vi "Global Log To String(Periodic Check).vi"(0 "Cross CSM Data":T3, 1 "Reset?":bool, 2 "Remove Immediately? (F)":bool, 3 "Time Format String":string="%<%H:%M:%S%3u>T", 9 "Settings":T2={"threashold(#/s)"=1.9, "Check Peroid(s)"=1.0}, 12 "Level (Normal)":T1) -> (4 "String":string, 10 "Periodic Info":string[](array[string]))   [LabVIEW 2017, in "Communicable State Machine.lvlib"]
uses:
  Communicable State Machine.lvlib
  _Support/Typedef/_CSM_GlobalLog_MSG.ctl
  _Support/Typedef/_CSM_Response Source Message.ctl
  _Support/Typedef/_CSM_GlobalLog_MSG_TYPE.ctl
  Periodic String Filter Setting.ctl
  _support/Periodic String Filter Level.ctl
  Periodic String Filter State.ctl
  _Shared/CSM Shared.lvlib
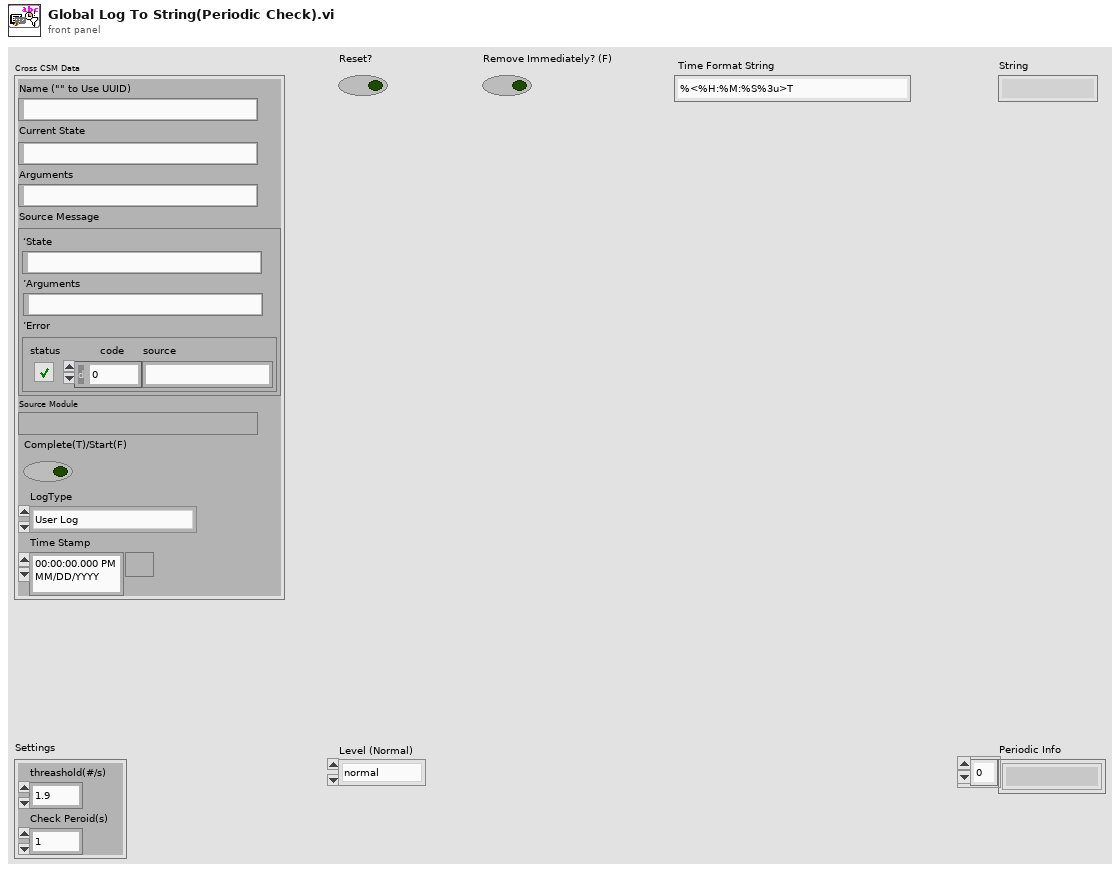
[diagram p1: front panel]
types:
  T1 = typedef "Communicable State Machine.lvlib/Periodic String Filter Level.ctl" = enum16{"normal", "L1", "L2", "L3", "L4"}
  T2 = typedef "Communicable State Machine.lvlib/Periodic String Filter Setting.ctl" = cluster{"threashold(#/s)":dbl, "Check Peroid(s)":dbl}
  T3 = typedef "Communicable State Machine.lvlib/_CSM_GlobalLog_MSG.ctl" = cluster{"Name (\"\" to Use UUID)":string, "Current State":string, "Arguments":string, "Source Message":T4, "Source Module":string, "Complete(T)/Start(F)":bool, "LogType":T5, "Time Stamp":timestamp}
  T4 = typedef "Communicable State Machine.lvlib/_CSM_Response Source Message.ctl" = cluster{"‘State":string, "’Arguments":string, "’Error":errorcluster}
  T5 = typedef "Communicable State Machine.lvlib/_CSM_GlobalLog_MSG_TYPE.ctl" = enum16{"User Log", "State Change", "Status", "Interrupt", "Register", "Unregister", "Error Log", "Module Created", "Module Destroyed", "Async Message", "No-Rep Async Message", "Sync Message"}
  T6 = typedef "Communicable State Machine.lvlib/Periodic String Filter State.ctl" = enum16{"Normal", "Remove All Filters"}
  T7 = typedef "Communicable State Machine.lvlib/Periodic String Filter Data.ctl" = cluster{"Keys":string[], "Count":i64[], "LastCheckT":timestamp[], "LastCheckN":i64[], "Filtered":cluster{"Keys":string[], "StartingCount":i64[], "entry":T8[]}}
  T8 = typedef "Communicable State Machine.lvlib/Periodic String Filter Info.ctl" = cluster{"String":string, "Count":i64, "since":timestamp, "param":string, "speed":dbl}
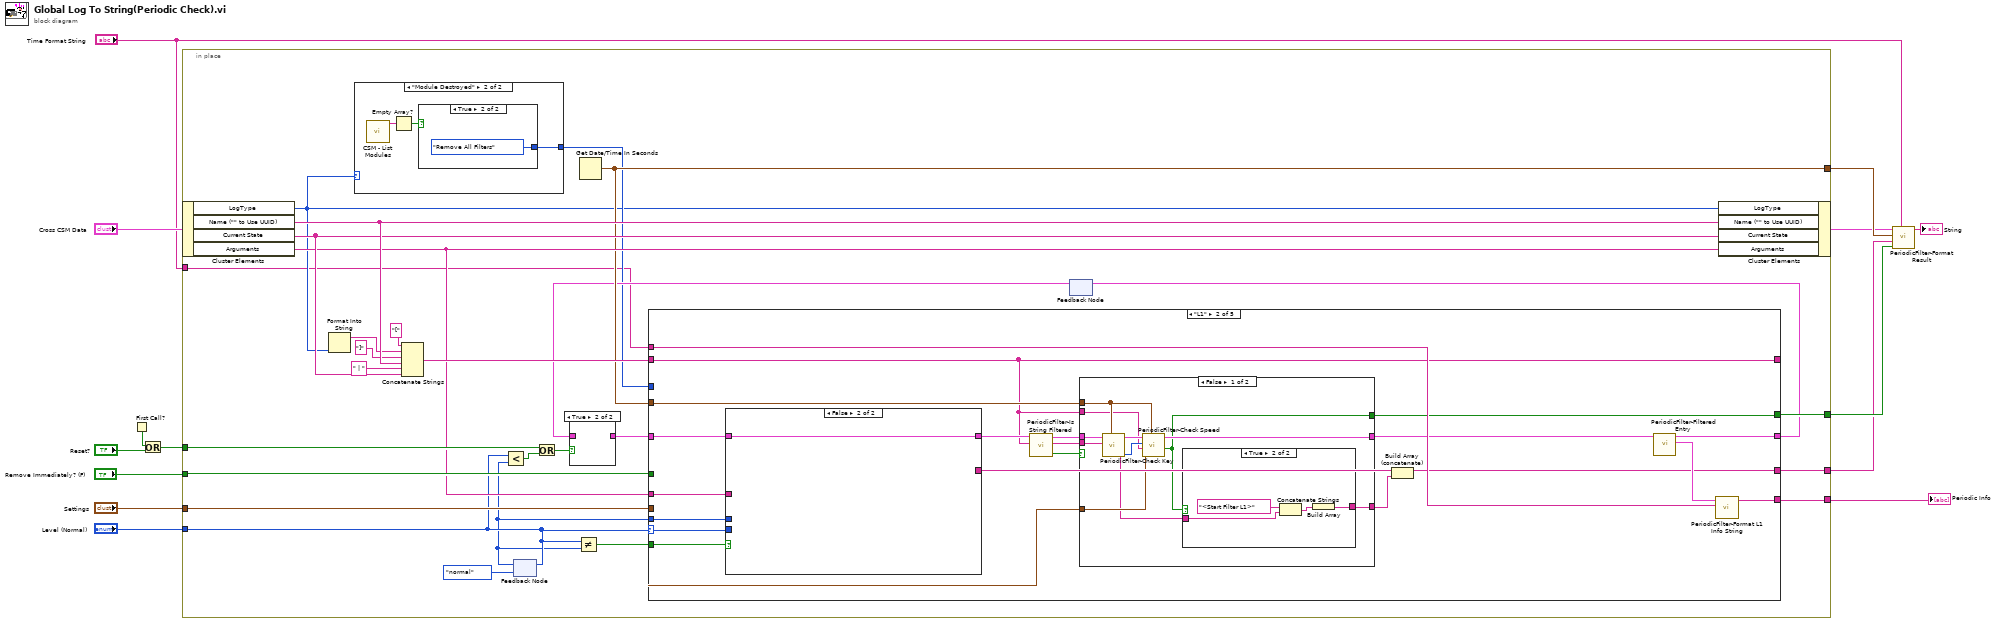
[diagram p0: block diagram]
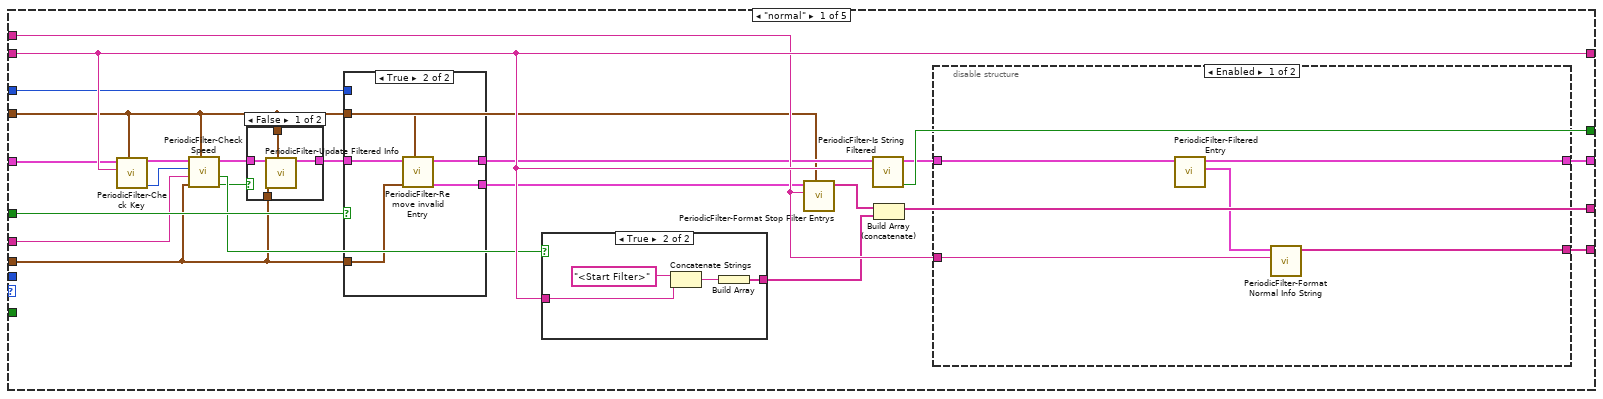
[diagram p4: hidden frame]
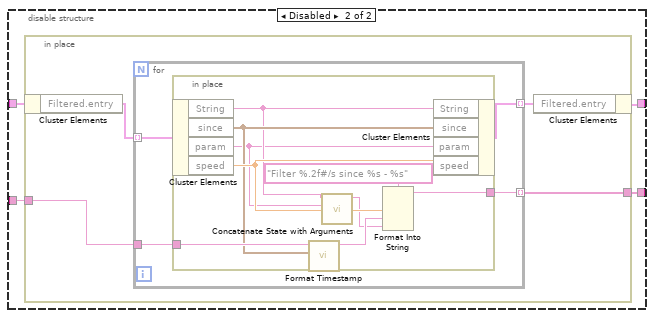
[diagram p6: hidden frame]
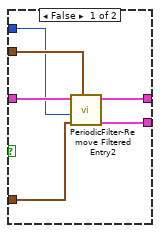
[diagram p7: hidden frame]
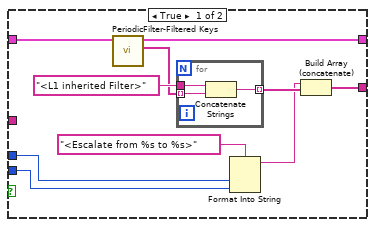
[diagram p11: hidden frame]
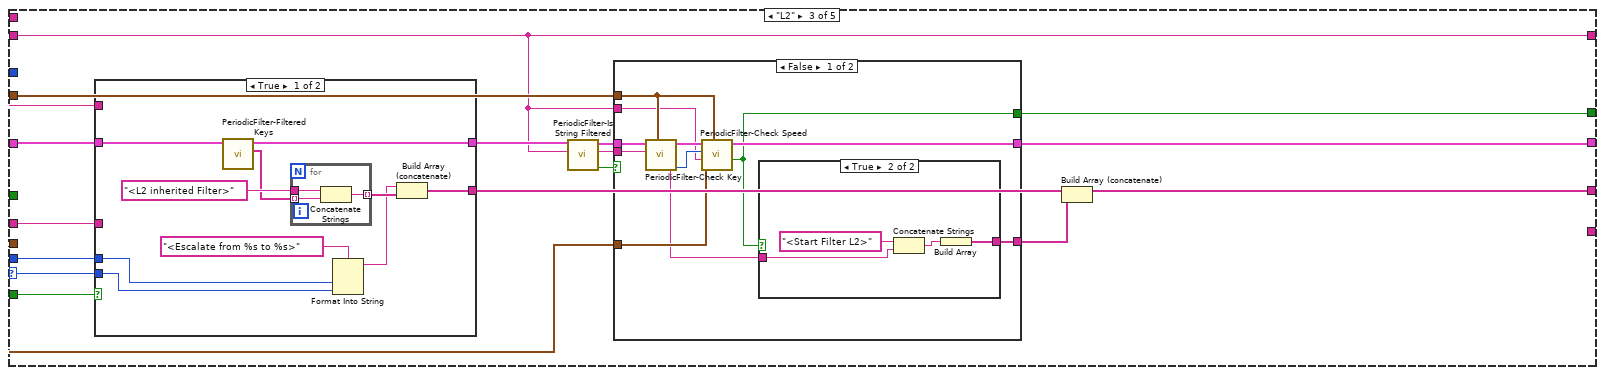
[diagram p12: hidden frame]
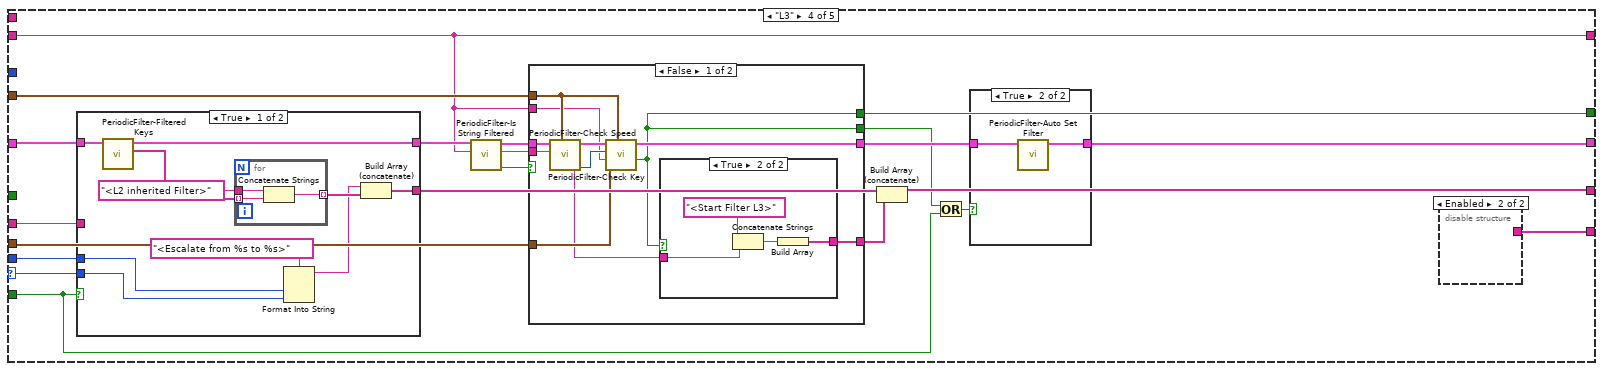
[diagram p16: hidden frame]
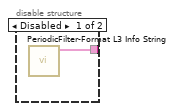
[diagram p17: hidden frame]
diagram:
  n1 = First Call?() -> (First Call?: T/F=w5:bool)
  n2 = Or(x=w5, y="Reset?") -> (x .or. y?=w6:bool)
  n3 = in-place "In Place Element Structure" {
    in-place-border: w6 -> [w38]
    in-place-border: [w36] -> w10
    in-place-border: "Remove Immediately? (F)" -> [w33]
    in-place-border: "Settings" -> [w32]
    in-place-border: "Level (Normal)" -> [w16]
    in-place-border: [w29] -> w9
    in-place-border: [w19] -> w1
    in-place-border: [w18] -> w4
    in-place-border: "Time Format String" -> [w17]
    n4 = in-place-cluster #1("Cross CSM Data") -> ("LogType"=w20:T5, "Name (\"\" to Use UUID)"=w41:string, "Current State"=w40:string, "Arguments"=w31:string)
    n5 = Format Into String(w20) -> (resulting string=w30:string)  [unwired: 3 in, 1 out]
    n6 = case shown="\"Module Destroyed\"" w20 {
      tunnel: [_ w42] -> w21
      frame "User Log", Default {
      }
      frame "Module Destroyed" {
        n7 = call "CSM - List Modules.vi"() -> ("Module Names"=w44:string[])  [unwired: 10 in, 1 out]
        n8 = Empty Array?(array=w44) -> (empty?=w43:bool)
        n9 = case shown="True" w43 {
          tunnel: [_ Periodic_String_Filter_State."Remove All Filters" ("State")] -> w42
          frame False {
          }
          frame True {
          }
        }
      }
    }
    n10 = Concatenate Strings("[" ("string"), w30, "]" ("string"), w41, " | " ("string"), w40) -> (w37:string)
    n11 = feedback #2(Periodic_String_Filter_Level."normal" ("Level(Normal)")) -> (w15:T1)
    n12 = Less?(x=w16, y=w15) -> (x < y?=w27:bool)
    n13 = feedback-in #2(w16) -> ()
    n14 = Or(x=w38, y=w27) -> (x .or. y?=w22:bool)
    n15 = Not Equal?(x=w16, y=w15) -> (x != y?=w26:bool)
    n16 = Get Date/Time In Seconds() -> (seconds since 1Jan1904=w29:timestamp)
    n17 = feedback #3() -> (w25:T7)  [unwired: 1 in]
    n18 = case shown="True" w22 {
      tunnel: [w278 _] -> w24
      tunnel: w25 -> [w278 _]
      frame False {
      }
      frame True {
      }
    }
    n19 = case shown="\"L1\"" w16 {
      selector: w16 -> [_ w115 w166 w213 _]
      tunnel: w37 -> [w68 w117 w168 w220 w273]
      tunnel: [w68 w117 w168 w220 w273] -> _
      tunnel: w32 -> [w48 w121 w172 w223 _]
      tunnel: w29 -> [w46 w122 w173 w224 _]
      tunnel: [w66 w128 w175 w219 w269] -> w23
      tunnel: w24 -> [w65 w135 w182 w233 w271]
      tunnel: [w64 w120 w171 w217 TRUE ("new filtered Item")] -> w36
      tunnel: w33 -> [w67 _ _ _ _]
      tunnel: w26 -> [_ w134 w181 w218 w270]
      tunnel: w31 -> [w63 w133 w180 w232 _]
      tunnel: w21 -> [w62 _ _ _ _]
      tunnel: [w61 w132 _ w231 _] -> w19
      tunnel: [w60 w119 w170 w222 w268] -> w18
      tunnel: w17 -> [w59 w131 _ _ _]
      tunnel: w15 -> [_ w116 w167 w214 _]
      frame "normal" {
        n20 = call "PeriodicFilter-Check Key.vi"("Seconds Since 1Jan1904 2"=w46, "Key"=w68, "Data In"=w65) -> ("Index"=w58:i32, "Data Out"=w57:T7)  [unwired: 7 in]
        n21 = call "PeriodicFilter-Check Speed.vi"("Seconds Since 1Jan1904"=w46, "Settings"=w48, "Parameter"=w63, "Index"=w58, "Data In"=w57) -> ("Over Threshold?"=w47:bool, "New Filtered Item"=w54:bool, "Data Out"=w56:T7)  [unwired: 4 in]
        n22 = case shown="False" w47 {
          tunnel: w56 -> [w72 w73]
          tunnel: [w71 w73] -> w55
          tunnel: w46 -> [w70 _]
          tunnel: w48 -> [w69 _]
          frame False {
            n23 = call "PeriodicFilter-Update Filtered Info.vi"("Seconds Since 1Jan1904"=w70, "Settings"=w69, "Data In"=w72) -> ("Data Out"=w71:T7)  [unwired: 8 in]
          }
          frame True {
          }
        }
        n24 = case shown="True" w67 {
          tunnel: w55 -> [w105 w110]
          tunnel: w46 -> [w104 w109]
          tunnel: [w103 w108] -> w53
          tunnel: [w102 w107] -> w52
          tunnel: w48 -> [w100 w106]
          tunnel: w62 -> [w101 _]
          frame False {
            n25 = call "PeriodicFilter-Remove Filtered Entry2.vi"("Seconds Since 1Jan1904 2"=w104, "Settings"=w100, "State"=w101, "Data In"=w105) -> ("Removed Info"=w102:T8[], "Data Out"=w103:T7)  [unwired: 6 in]
          }
          frame True {
            n26 = call "PeriodicFilter-Remove invalid Entry.vi"("Seconds Since 1Jan1904 2"=w109, "Settings"=w106, "Data In"=w110) -> ("Removed Info"=w107:T8[], "Data Out"=w108:T7)  [unwired: 7 in]
          }
        }
        n27 = case shown="True" w54 {
          tunnel: [_ w114] -> w50
          tunnel: w68 -> [_ w112]
          frame False {
          }
          frame True {
            n28 = Concatenate Strings("<Start Filter>" ("Current State"), w112) -> (w111:string)
            n29 = Build Array(w111) -> (w114:string[])
          }
        }
        n30 = call "PeriodicFilter-Format Stop Filter Entrys.vi"("Seconds Since 1Jan1904 2"=w46, "Time Format String"=w59, "Removed Info"=w52) -> ("Array"=w49:string[])  [unwired: 8 in]
        n31 = call "PeriodicFilter-Is String Filtered.vi"("Input String"=w68, "Data In"=w53) -> ("Filtered"=w64:bool, "Data Out"=w51:T7)  [unwired: 7 in, 1 out]
        n32 = Build Array (concatenate)(w49, w50) -> (w60:string[])
        n33 = disable-structure shown="Enabled" {
          disable-tunnel: [w78 w81] -> w66
          disable-tunnel: [w77 w79] -> w61
          disable-tunnel: w59 -> [w76 w80]
          disable-tunnel: w51 -> [w75 w82]
          frame Enabled {
            n34 = call "PeriodicFilter-Filtered Entry.vi"("Data In"=w75) -> ("Entry"=w74:T8[], "Data Out"=w78:T7)  [unwired: 9 in]
            n35 = call "PeriodicFilter-Format Normal Info String.vi"("Time Format String"=w76, "Removed Info"=w74) -> ("Array"=w77:string[])  [unwired: 9 in]
          }
          frame Disabled {
            n36 = in-place {
              in-place-border: w80 -> [w85]
              in-place-border: [w84] -> w79
              n37 = in-place-cluster #4(w82) -> ("Filtered.entry"=w86:T8[])
              n38 = for {
                tunnel: w86 -> [w88] mode=indexing
                tunnel: [w90] -> w84 mode=indexing
                tunnel: w85 -> [w89]
                tunnel: [w87] -> w83 mode=indexing
                n39 = in-place {
                  in-place-border: [w99] -> w90
                  in-place-border: w89 -> [w96]
                  n40 = in-place-cluster #5(w88) -> ("String"=w93:string, "since"=w94:timestamp, "param"=w91:string, "speed"=w95:dbl)
                  n41 = call "Format Timestamp.vi"("Timestamp"=w94, "Format String"=w96) -> ("String"=w97:string)  [unwired: 9 in]
                  n42 = call "Concatenate State with Arguments.vi"("Arguments"=w91, "State"=w93) -> ("State With Arguements"=w92:string)  [unwired: 9 in]
                  n43 = Format Into String(format string="Filter %.2f#/s since %s - %s", w95, w97, w92) -> (resulting string=w99:string)  [unwired: 2 in, 1 out]
                  n44 = in-place-cluster #5("String"=w93, "since"=w94, "param"=w91, "speed"=w95) -> (w87:T8)
                }
              }
              n45 = in-place-cluster #4("Filtered.entry"=w83) -> (w81:T7)
            }
          }
        }
      }
      frame "L1" {
        n46 = case shown="False" w134 {
          tunnel: w135 -> [w161 w165]
          tunnel: [w156 w165] -> w123
          tunnel: [w157 _] -> w130
          tunnel: w133 -> [_ _]
          tunnel: w116 -> [w154 _]
          tunnel: w115 -> [w153 _]
          frame True {
            n47 = call "PeriodicFilter-Filtered Keys.vi"("Data In"=w161) -> ("Filtered Keys"=w159:string[], "Data Out"=w156:T7)  [unwired: 9 in]
            n48 = for {
              tunnel: w159 -> [w164] mode=indexing
              tunnel: [w163] -> w158 mode=indexing
              tunnel: "<L1 inherited Filter>" ("Current State") -> [w162]
              n49 = Concatenate Strings(w162, w164) -> (w163:string)
            }
            n50 = Format Into String(format string="<Escalate from %s to %s>" ("Current State"), w154, w153) -> (resulting string=w152:string)  [unwired: 2 in, 1 out]
            n51 = Build Array (concatenate)(w152, w158) -> (w157:string[])
          }
          frame False {
          }
        }
        n52 = call "PeriodicFilter-Is String Filtered.vi"("Input String"=w117, "Data In"=w123) -> ("Filtered"=w125:bool, "Input String (Dup)"=w127:string, "Data Out"=w126:T7)  [unwired: 7 in]
        n53 = case shown="False" w125 {
          selector: w125 -> [_ w150]
          tunnel: w126 -> [w143 w151]
          tunnel: [w142 w151] -> w124
          tunnel: w122 -> [w141 _]
          tunnel: w127 -> [w136 _]
          tunnel: [w140 _] -> w118
          tunnel: [w139 w150] -> w120
          tunnel: w121 -> [w138 _]
          tunnel: w117 -> [w137 _]
          frame False {
            n54 = call "PeriodicFilter-Check Key.vi"("Seconds Since 1Jan1904 2"=w141, "Key"=w136, "Data In"=w143) -> ("Index"=w144:i32, "Data Out"=w145:T7)  [unwired: 7 in]
            n55 = call "PeriodicFilter-Check Speed.vi"("Seconds Since 1Jan1904"=w141, "Settings"=w138, "Parameter"=w137, "Index"=w144, "Data In"=w145) -> ("New Filtered Item"=w139:bool, "Data Out"=w142:T7)  [unwired: 4 in, 1 out]
            n56 = case shown="True" w139 {
              tunnel: [_ w146] -> w140
              tunnel: w136 -> [_ w149]
              frame False {
              }
              frame True {
                n57 = Concatenate Strings("<Start Filter L1>" ("Current State"), w149) -> (w147:string)
                n58 = Build Array(w147) -> (w146:string[])
              }
            }
          }
          frame True {
          }
        }
        n59 = Build Array (concatenate)(w130, w118) -> (w119:string[])
        n60 = call "PeriodicFilter-Filtered Entry.vi"("Data In"=w124) -> ("Entry"=w129:T8[], "Data Out"=w128:T7)  [unwired: 9 in]
        n61 = call "PeriodicFilter-Format L1 Info String.vi"("Time Format String"=w131, "Entry"=w129) -> ("Array"=w132:string[])  [unwired: 9 in]
      }
      frame "L2" {
        n62 = case shown="True" w181 {
          tunnel: w182 -> [w208 w212]
          tunnel: [w203 w212] -> w174
          tunnel: w168 -> [_ _]
          tunnel: [w204 _] -> w179
          tunnel: w180 -> [_ _]
          tunnel: w167 -> [w201 _]
          tunnel: w166 -> [w200 _]
          frame True {
            n63 = call "PeriodicFilter-Filtered Keys.vi"("Data In"=w208) -> ("Filtered Keys"=w206:string[], "Data Out"=w203:T7)  [unwired: 9 in]
            n64 = for {
              tunnel: w206 -> [w211] mode=indexing
              tunnel: [w210] -> w205 mode=indexing
              tunnel: "<L2 inherited Filter>" ("Current State") -> [w209]
              n65 = Concatenate Strings(w209, w211) -> (w210:string)
            }
            n66 = Format Into String(format string="<Escalate from %s to %s>" ("Current State"), w201, w200) -> (resulting string=w199:string)  [unwired: 2 in, 1 out]
            n67 = Build Array (concatenate)(w199, w205) -> (w204:string[])
          }
          frame False {
          }
        }
        n68 = call "PeriodicFilter-Is String Filtered.vi"("Input String"=w168, "Data In"=w174) -> ("Filtered"=w176:bool, "Input String (Dup)"=w178:string, "Data Out"=w177:T7)  [unwired: 7 in]
        n69 = case shown="False" w176 {
          selector: w176 -> [_ w197]
          tunnel: w177 -> [w190 w198]
          tunnel: [w189 w198] -> w175
          tunnel: w173 -> [w188 _]
          tunnel: w178 -> [w183 _]
          tunnel: [w187 _] -> w169
          tunnel: [w186 w197] -> w171
          tunnel: w172 -> [w185 _]
          tunnel: w168 -> [w184 _]
          frame False {
            n70 = call "PeriodicFilter-Check Key.vi"("Seconds Since 1Jan1904 2"=w188, "Key"=w183, "Data In"=w190) -> ("Index"=w191:i32, "Data Out"=w192:T7)  [unwired: 7 in]
            n71 = call "PeriodicFilter-Check Speed.vi"("Seconds Since 1Jan1904"=w188, "Settings"=w185, "Parameter"=w184, "Index"=w191, "Data In"=w192) -> ("New Filtered Item"=w186:bool, "Data Out"=w189:T7)  [unwired: 4 in, 1 out]
            n72 = case shown="True" w186 {
              tunnel: [_ w193] -> w187
              tunnel: w183 -> [_ w196]
              frame False {
              }
              frame True {
                n73 = Concatenate Strings("<Start Filter L2>" ("Current State"), w196) -> (w194:string)
                n74 = Build Array(w194) -> (w193:string[])
              }
            }
          }
          frame True {
          }
        }
        n75 = Build Array (concatenate)(w179, w169) -> (w170:string[])
      }
      frame "L3" {
        n76 = case shown="True" w218 {
          tunnel: w233 -> [w260 w267]
          tunnel: [w259 w267] -> w225
          tunnel: [w263 _] -> w230
          tunnel: w232 -> [_ _]
          tunnel: w214 -> [w256 _]
          tunnel: w213 -> [w255 _]
          frame True {
            n77 = call "PeriodicFilter-Filtered Keys.vi"("Data In"=w260) -> ("Filtered Keys"=w262:string[], "Data Out"=w259:T7)  [unwired: 9 in]
            n78 = for {
              tunnel: w262 -> [w266] mode=indexing
              tunnel: [w265] -> w258 mode=indexing
              tunnel: "<L2 inherited Filter>" ("Current State") -> [w264]
              n79 = Concatenate Strings(w264, w266) -> (w265:string)
            }
            n80 = Format Into String(format string="<Escalate from %s to %s>" ("Current State"), w256, w255) -> (resulting string=w254:string)  [unwired: 2 in, 1 out]
            n81 = Build Array (concatenate)(w254, w258) -> (w263:string[])
          }
          frame False {
          }
        }
        n82 = call "PeriodicFilter-Is String Filtered.vi"("Input String"=w220, "Data In"=w225) -> ("Filtered"=w227:bool, "Input String (Dup)"=w229:string, "Data Out"=w228:T7)  [unwired: 7 in]
        n83 = case shown="False" w227 {
          selector: w227 -> [_ w252]
          tunnel: w228 -> [w245 w253]
          tunnel: [w244 w253] -> w226
          tunnel: w224 -> [w243 _]
          tunnel: w229 -> [w239 _]
          tunnel: [w242 _] -> w221
          tunnel: [w238 w252] -> w217
          tunnel: w223 -> [w241 _]
          tunnel: w220 -> [w240 _]
          tunnel: [w238 _] -> w215
          frame False {
            n84 = call "PeriodicFilter-Check Key.vi"("Seconds Since 1Jan1904 2"=w243, "Key"=w239, "Data In"=w245) -> ("Index"=w246:i32, "Data Out"=w247:T7)  [unwired: 7 in]
            n85 = call "PeriodicFilter-Check Speed.vi"("Seconds Since 1Jan1904"=w243, "Settings"=w241, "Parameter"=w240, "Index"=w246, "Data In"=w247) -> ("New Filtered Item"=w238:bool, "Data Out"=w244:T7)  [unwired: 4 in, 1 out]
            n86 = case shown="True" w238 {
              tunnel: [_ w248] -> w242
              tunnel: w239 -> [_ w251]
              frame False {
              }
              frame True {
                n87 = Concatenate Strings("<Start Filter L3>" ("Current State"), w251) -> (w249:string)
                n88 = Build Array(w249) -> (w248:string[])
              }
            }
          }
          frame True {
          }
        }
        n89 = Build Array (concatenate)(w230, w221) -> (w222:string[])
        n90 = Or(x=w215, y=w218) -> (x .or. y?=w216:bool)
        n91 = case shown="True" w216 {
          tunnel: w226 -> [w235 w237]
          tunnel: [w235 w236] -> w219
          frame False {
          }
          frame True {
            n92 = call "PeriodicFilter-Auto Set Filter.vi"("Data In"=w237) -> ("Data Out"=w236:T7)  [unwired: 10 in]
          }
        }
        n93 = disable-structure shown="Enabled" {
          disable-tunnel: [w234 _] -> w231
          frame Disabled {
            n94 = call "PeriodicFilter-Format L3 Info String.vi"() -> ("Array"=w234:string[])  [unwired: 11 in]
          }
          frame Enabled {
          }
        }
      }
      frame Default {
        n95 = case shown="True" w270 {
          tunnel: w271 -> [w274 w277]
          tunnel: [w274 w277] -> w269
          tunnel: [w275 _] -> w268
          frame True {
            n96 = Build Array("<Escalate from Top Level, All messages are filtered.>" ("Current State")) -> (w275:string[])
          }
          frame False {
          }
        }
      }
    }
    n97 = feedback-in #3(w23) -> ()
    n98 = in-place-cluster #1("LogType"=w20, "Name (\"\" to Use UUID)"=w41, "Current State"=w40, "Arguments"=w31) -> (w8:T3)
  }
  "Periodic Info" <- w1
  n99 = call "PeriodicFilter-Format Result.vi"("Time Format String"="Time Format String", "Filtered"=w10, "Additional Info"=w4, "Current Time"=w9, "Cross CSM Data In"=w8) -> ("States"=→"String":string)  [unwired: 6 in]
